vi "Thresholding.vi"(7 "Threshold":u16, 11 "RAW SICK Data":T1) -> (2 "Boolean array":bool[](array[boolean]))   [LabVIEW 2009]
doc: "Thresholding, True means passable"
uses:
  TypeDefs/Sensor Typedefs/SICK Array.ctl
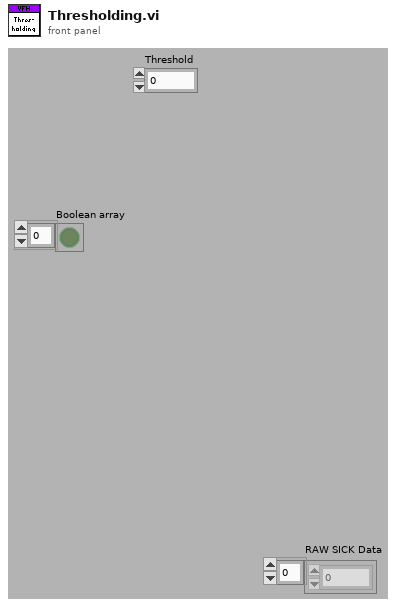
[diagram p1: front panel]
types:
  T1 = typedef "SICK Array.ctl" = u16[]
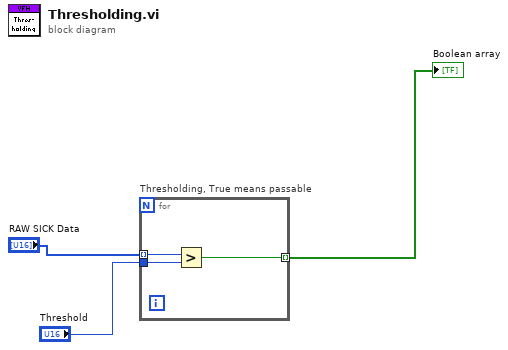
[diagram p0: block diagram]
diagram:
  n1 = for "Thresholding, True means passable" {
    tunnel: "RAW SICK Data" -> [w6] mode=indexing
    tunnel: "Threshold" -> [w5]
    tunnel: [w4] -> w2 mode=indexing
    n2 = Greater?(x=w6, y=w5) -> (0:w4:bool)
  }
  "Boolean array" <- w2
